vi "Logging Configuration.vi"() -> ()   [LabVIEW 2019, in "Logger.lvlib" / "Logger.lvclass"]
uses:
  Logger.lvclass
  Type Defs/Logging Level.ctl
panel:
  in  "Logging Level":T1=enum."Trace"
  in  "Queue Name":string
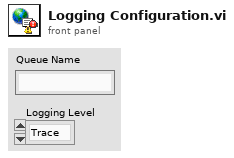
[diagram p1: front panel]
types:
  T1 = typedef "Logger.lvlib/Logger.lvclass/Logging Level.ctl" = enum16{"Error", "Warning", "Info", "Trace"}
diagram:
